vi "host_test.vi"   [LabVIEW 2010]
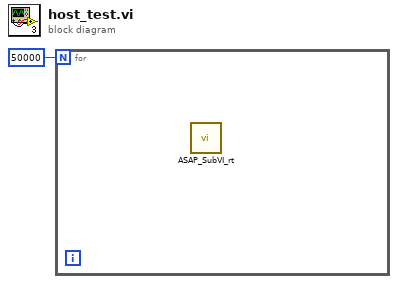
[diagram p0: block diagram]
diagram:
  n1 = for {
    N: 50000 -> [_]
    n2 = call "ASAP_SubVI_rt.vi"() -> ()  [unwired: 4 in, 8 out]
  }
